vi "cRIO VI parameters.vi"() -> ()   [LabVIEW 2024]
panel:
  in  "RT Stop refnum":refnum<k21>="ni.var.psp://NI-cRIO-9063/network varibles/RT Stop"
  in  "Data buffer size refnum":refnum<k21>="ni.var.psp://NI-cRIO-9063/network varibles/Data buffer size"
  in  "cRIO IP":string="//172.22.11.2"
  in  "Data buffer size":i32=1000
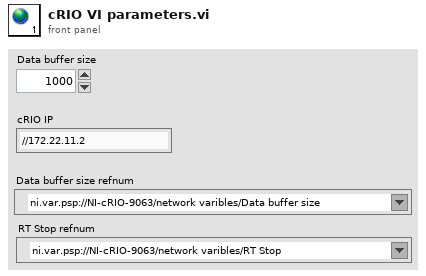
[diagram p1: front panel]
diagram:
